vi "Update Event Queue Nested.vi"(9 "Insert (T) or Remove (F)":bool, 10 "Queue Nested":map{string, refnum<data-value>}(c390), 11 "jettl Queue Actor in":refnum<class "jettl Queue Actor.lvclass">) -> (3 "jettl Queue Actor out":refnum<class "jettl Queue Actor.lvclass">)   [LabVIEW 2021, in "jettl.lvlib" / "jettl Queue Actor.lvclass"]
uses:
  jettl Queue Actor.lvclass
  Actor/Msg/Msg.lvclass
  Actor/Msgs/Update Queue Nested/Update Queue Nested Msg/Update Queue Nested Msg.lvclass
  C:/git/jettl/src/Actor/Msg/Msg.lvclass
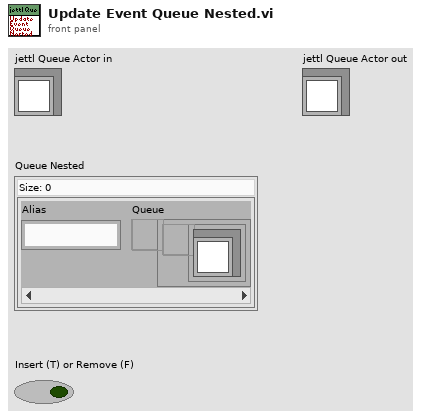
[diagram p1: front panel]
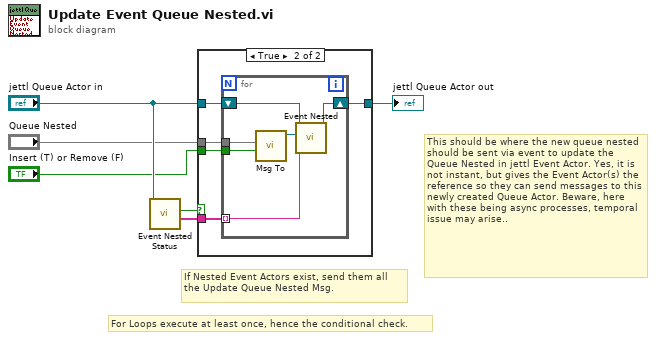
[diagram p0: block diagram]
diagram:
  # "This should be where the new queue nested should be sent via event to update the Queue Nested in jettl Event Actor. Yes, it is not instant, but gives the Event Actor(s) the reference so they can send messages to this newly created Queue Actor. Beware, here with these being async processes, temporal issue may arise.."
  # "If Nested Event Actors exist, send them all the Update Queue Nested Msg."
  # "For Loops execute at least once, hence the conditional check."
  n1 = call-dynamic "Event Nested Status.vi"("jettl Queue Actor in"="jettl Queue Actor in") -> ("Event Nested Aliases"=w5:string[], "Any Exist?"=w6:bool)  [unwired: 8 in, 1 out]
  n2 = case shown="True" w6 {
    tunnel: [w7 w12] -> w3
    tunnel: "jettl Queue Actor in" -> [w7 w11]
    tunnel: w5 -> [_ w10]
    tunnel: "Queue Nested" -> [_ w9]
    tunnel: "Insert (T) or Remove (F)" -> [_ w8]
    frame False {
    }
    frame True {
      n3 = for {
        tunnel: w10 -> [w16] mode=indexing
        shift-right: [w17] -> w12
        shift-left: w11 -> [w18]
        tunnel: w9 -> [w15]
        tunnel: w8 -> [w13]
        n4 = call "Msg To.vi"("Insert (T) or Remove (F)"=w13, "Queue Nested"=w15) -> ("Update Queue Nested Msg out"=w14:refnum<class "Update Queue Nested Msg.lvclass">)  [unwired: 9 in]
        n5 = call-dynamic "Event Nested.vi"("Alias"=w16, "Msg"=w14, "jettl Queue Actor in"=w18) -> ("jettl Queue Actor out"=w17:refnum<class "jettl Queue Actor.lvclass">)  [unwired: 8 in]
      }
    }
  }
  "jettl Queue Actor out" <- w3
